vi "update-tree-signal-values.vi"(8 "error in (no error)":errorcluster, 9 "CAN frame":T1 {"payload" format="%x"; "timestamp" format="%<%.7X\n%x>T"; "type" items=["CAN Data"=0, "CAN Remote"=1, "CAN Bus Error"=2, "J1939 Data"=192, "Delay"=224, "Log Trigger"=225, "Start Trigger"=226]; "identifier" format="%x"}, 10 "TAGS":string[](array[string]), 11 "dbc in":refnum<class "dbc.lvclass">) -> (0 "error out":errorcluster, 3 "dbc out":refnum<class "dbc.lvclass">)   [LabVIEW 2015, in "dbc.lvclass"]
uses:
  dbc.lvclass
  <vilib>/xnet/xnet.llb/XNET Frame CAN.ctl
  <vilib>/xnet/xnet.llb/XNET Frame Type CAN.ctl
  dbc.lvclass/dbc.ctl
  <resource>/objmgr/xnet.rc
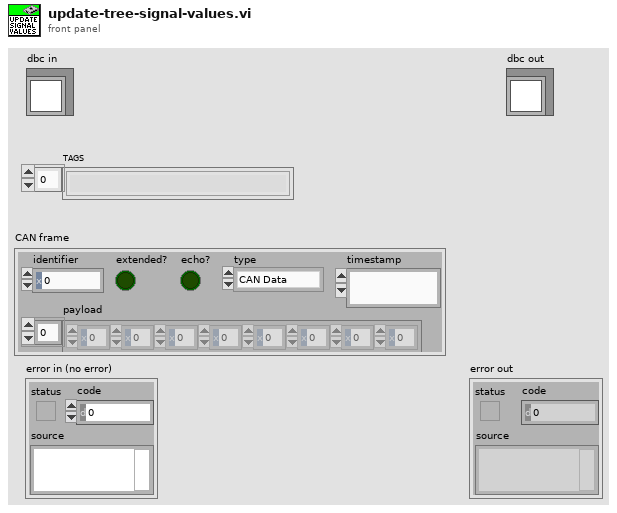
[diagram p1: front panel]
types:
  T1 = typedef "XNET Frame CAN.ctl" = cluster{"timestamp":timestamp, "payload":u8[], "identifier":u32, "type":T2, "extended?":bool, "echo?":bool}
  T2 = typedef "XNET Frame Type CAN.ctl" = u8
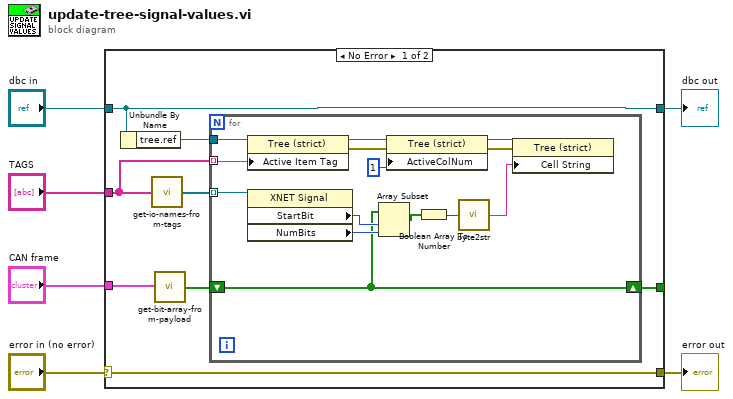
[diagram p0: block diagram]
diagram:
  n1 = case shown="No Error" "error in (no error)" {
    selector: "error in (no error)" -> [w11 w30]
    tunnel: [w11 w30] -> w5
    tunnel: [w8 w29] -> w3
    tunnel: "dbc in" -> [w8 w29]
    tunnel: "TAGS" -> [w10 _]
    tunnel: "CAN frame" -> [w9 _]
    tunnel: [w12 _] -> _
    frame No Error {
      n2 = Unbundle By Name(w8) -> ("tree.ref"=w7:refnum<vi>)
      n3 = call "get-io-names-from-tags.vi"("tags"=w10) -> ("Array"=w13:refnum<k21>[])  [unwired: 4 in]
      n4 = call "get-bit-array-from-payload.vi"("CAN frame"=w9) -> ("Array"=w14:bool[])  [unwired: 4 in]
      n5 = for {
        tunnel: w13 -> [w28] mode=indexing
        shift-right: [w25] -> w12
        shift-left: w14 -> [w25]
        tunnel: w10 -> [w17] mode=indexing
        tunnel: w7 -> [w16]
        n6 = property class="Tree (strict)"(reference=w16, "Active Item Tag"=w17) -> (reference out=w20:refnum<vi>, error out=w19:errorcluster)  [unwired: 1 in]
        n7 = property class="XNET Signal"(reference=w28) -> ("StartBit"=w26:u32, "NumBits"=w27:u32)  [unwired: 1 in, 2 out]
        n8 = Array Subset(array=w25, index=w26, length=w27) -> (w24:bool[])
        n9 = property class="Tree (strict)"(reference=w20, error in=w19, "ActiveColNum"=1 ("Active Cell:Active Column Number")) -> (reference out=w22:refnum<vi>, error out=w18:errorcluster)
        n10 = Boolean Array To Number(Boolean array=w24) -> (number=w23:u32)
        n11 = call "byte2str.vi"("byte"=w23) -> ("String"=w15:string)  [unwired: 4 in]
        n12 = property class="Tree (strict)"(reference=w22, error in=w18, "Cell String"=w15) -> ()  [unwired: 2 out]
      }
    }
    frame Error {
    }
  }
  "error out" <- w5
  "dbc out" <- w3
